vi "ImportFileInWaveformList.vi"(1 "Select  File Name (Absolute Path) to Import  from AWG's Files System":path, 3 "error in (no error)":errorcluster, 4 "Specify the  Waveform Type":u16(ring) items=["Analog", "Digitals"], 5 "Set the Waveform Name":string, 6 "VISA resource name":refnum<visa-resource-name>) -> (0 "error out":errorcluster, 2 "VISA resource name out":refnum<visa-resource-name>)   [LabVIEW 2020, in "Active Technologies AWG3000.lvlib"]
uses:
  Active Technologies AWG3000.lvlib
panel:
  # "Only .txt, .trc or .zip format is allowed.\nNote: for Drive C  is allowed import a waveform only from the default folder or its subdirectories. \nNo limitation for the other drivers.\nTo know the default directory, run GetDefaultDriveCFolder.vi."
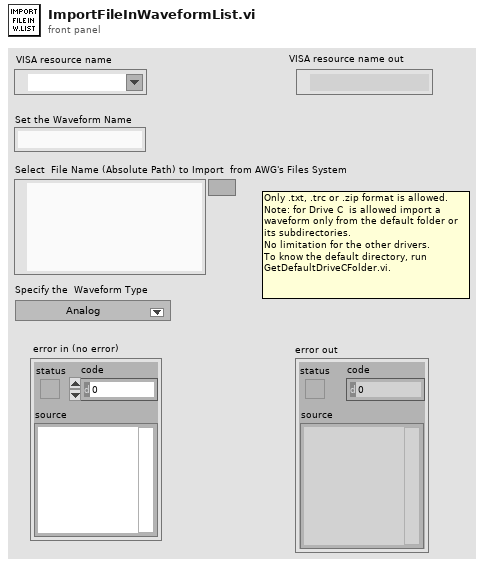
[diagram p1: front panel]
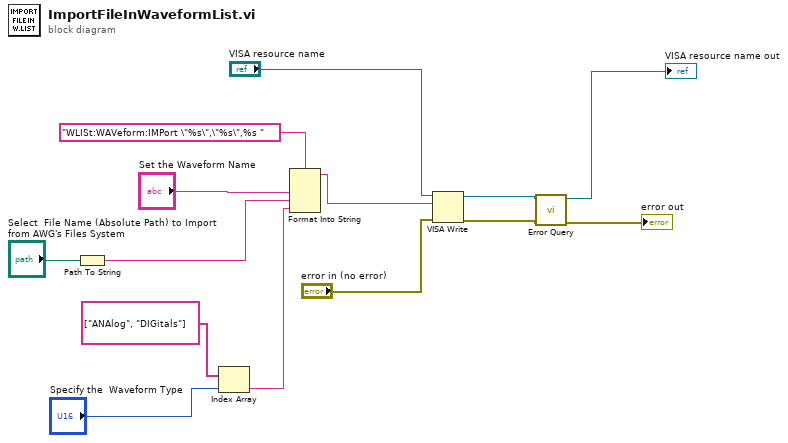
[diagram p0: block diagram]
diagram:
  n1 = Path To String(path="Select  File Name (Absolute Path) to Import  from AWG's Files System") -> (string=w8:string)
  n2 = Index Array(array=string[] ["ANAlog", "DIGitals"], index="Specify the  Waveform Type") -> (element=w2:string)
  n3 = Format Into String(format string="WLISt:WAVeform:IMPort \"%s\",\"%s\",%s " ("write buffer"), "Set the Waveform Name", w8, w2) -> (resulting string=w1:string)  [unwired: 2 in, 1 out]
  n4 = VISA Write(VISA resource name="VISA resource name", write buffer=w1, error in (no error)="error in (no error)") -> (VISA resource name out=w6:refnum<visa-resource-name>, error out=w5:errorcluster)  [unwired: 1 out]
  n5 = call "Error Query.vi"("error in (no error)"=w5, "VISA resource name"=w6) -> ("error out"=→"error out":errorcluster, "VISA resource name out"=→"VISA resource name out":refnum<visa-resource-name>)  [unwired: 6 in, 2 out]
